vi "Read from Hardware.vi"(8 "error in":errorcluster, 10 "Values in":dbl[](array[numeric]), 11 "AIM ARINC-429 Rx Execution Unit in":refnum<class "Rx Execution Unit.lvclass">) -> (0 "error out":errorcluster, 2 "Values out":dbl[](array[numeric]), 3 "AIM ARINC-429 Rx Execution Unit out":refnum<class "Rx Execution Unit.lvclass">)   [LabVIEW 2020, in "AIM ARINC 429 Engine.lvlib" / "Implementation.lvlib" / "Rx Execution Unit.lvclass"]
uses:
  Rx Execution Unit.lvclass
  Execution Unit/Execution Unit.lvclass
  Hardware API/AIM ARINC 429 Hardware API.lvlib
  Custom Device/Custom Device.lvlib
  <instrlib>/AIM GmbH/ARINC-429/AIM429LV.lvlib
  C:/Git/niveristand-aim-arinc429-custom-device/Source/Custom Device Support/Engine/Implementation/Execution Unit/Execution Unit.lvclass
  C:/Git/niveristand-aim-arinc429-custom-device/Source/Custom Device Support/Engine/Interfaces/Execution Unit/Execution Unit.lvclass
  C:/Git/niveristand-aim-arinc429-custom-device/Source/Custom Device Support/Engine/Implementation/Rx Execution Unit/Rx Execution Unit.lvclass
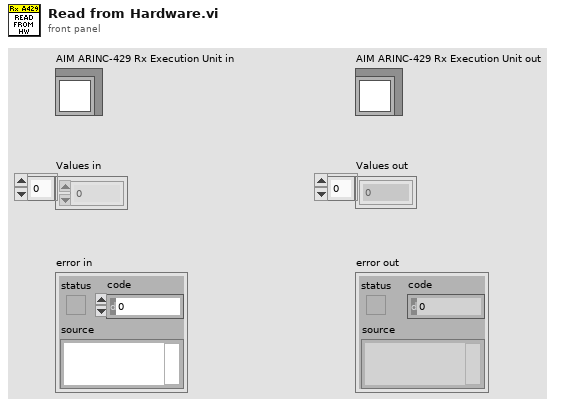
[diagram p1: front panel]
types:
  T1 = cluster{"hardware channel":u8, "label":u8, "SDI":u8}
  T2 = cluster{"gap":i16, "parity":i16, "long word":i16, "bit timing":i16, "timeout":i16}
  T3 = map{cluster{"hardware channel":u8, "label":u8, "SDI":u8}, cluster{"data word":u32, "time stamp":dbl}}
  T4 = typedef "AIM ARINC 429 Engine.lvlib/Custom Device.lvlib/Hardware Handles.ctl" = cluster{"module":u8}
  T5 = typedef "RT Hardware Channel Settings.ctl" = cluster{"channel #":u16, "channel handle":u64, "labels settings for RT":T6[]}
  T6 = typedef "RT Label Settings.ctl" = cluster{"Name":string, "xmlName":string, "label":T7, "transfer period":u32, "SDI_Enabled":bool, "SDI":u8, "parameter driver data":T8, "transfer type":T12, "has timestamp?":bool, "Label Disable/Trigger Channel Reference":T11, "Message Handle":u64, "Initialized?":bool, "Word Initial Raw Value":u32, "Label Timestamp Channel Data Reference":T13, "disabled":bool}
  T7 = typedef "Label.ctl" = u8
  T8 = typedef "RT Parameters.ctl" = cluster{"parameter definitions":T9[], "Tx parameter refs":T11[]}
  T9 = typedef "Parameter Definition.ctl" = cluster{"start index":i32, "size":i32, "encoding":T10, "signed":bool, "scale multiplier":dbl, "scale offset":dbl}
  T10 = typedef "Encoding and Decoding.lvlib/Encoding.ctl" = enum16{"BNR", "BCD", "Discrete"}
  T11 = typedef "Custom Device API.lvlib/Custom Device Item Ref.ctl" = u64
  T12 = typedef "Transfer Type.ctl" = enum16{"Scheduled", "Acyclic", "Block", "Strobe"}
  T13 = typedef "Custom Device API.lvlib/Data Reference.ctl" = i32
  T14 = cluster{"gap":bool, "parity":bool, "long word":bool, "bit timing":bool, "timeout":bool}
  T15 = typedef "Map of Identifiers to Indexes.ctl" = map{cluster{"Port":u8, "Label":u8, "SDI":u8}, cluster{"channel index":i32, "label index":i32, "start index":i32, "parameters":i32, "timestamp index":i32}}
  T16 = cluster{"receiving":T13, "specific errors":cluster{"gap":T13, "parity":T13, "long word ":T13, "bit timing":T13, "timeout":T13}}
  T17 = cluster{"receiving":dbl, "specific errors":cluster{"gap":dbl, "parity":dbl, "long word ":dbl, "bit timing":dbl, "timeout":dbl}}
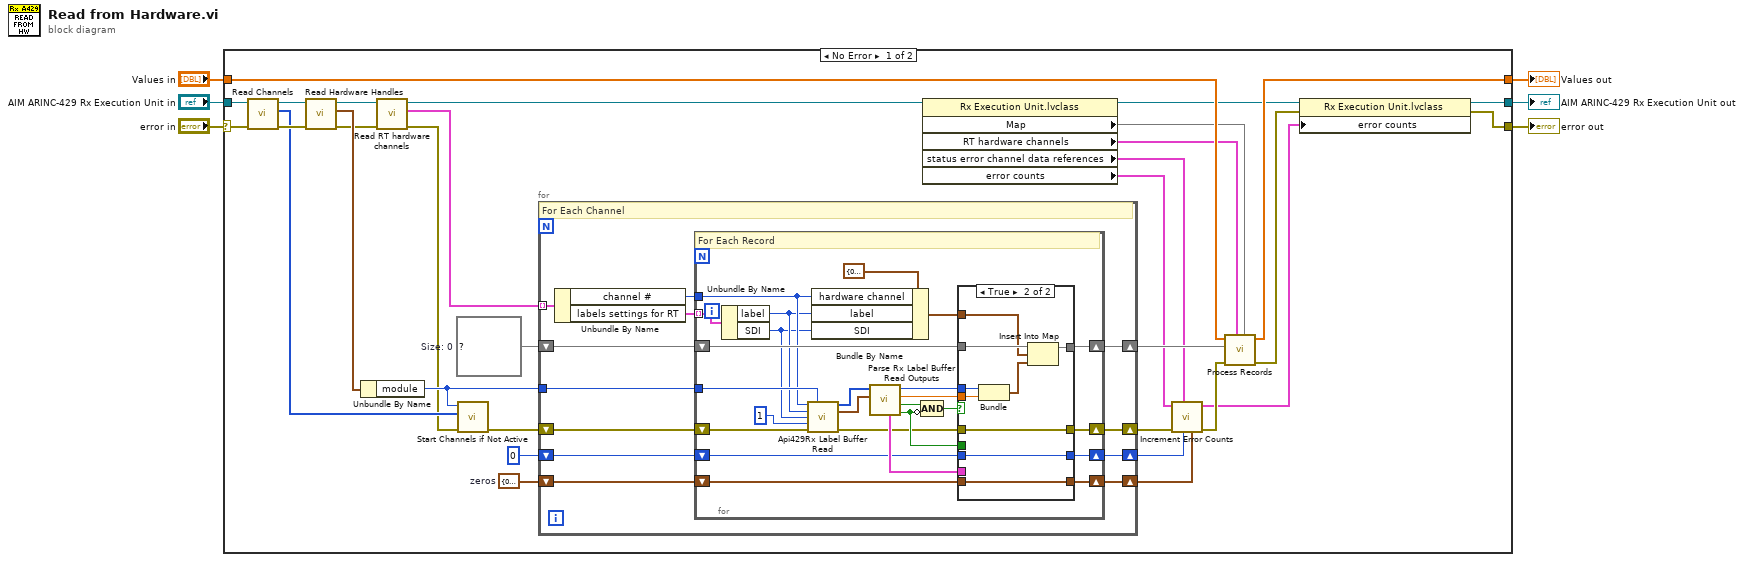
[diagram p0: block diagram]
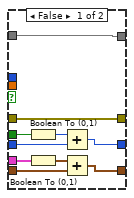
[diagram p2: hidden frame]
diagram:
  n1 = case shown="No Error" "error in" {
    selector: "error in" -> [w31 w96]
    tunnel: [w36 w97] -> w5
    tunnel: "AIM ARINC-429 Rx Execution Unit in" -> [w32 w97]
    tunnel: [w7 w96] -> w3
    tunnel: [w35 w95] -> w2
    tunnel: "Values in" -> [w34 w95]
    frame No Error {
      w16 = T2 {"gap"=0, "parity"=0, "long word"=0, "bit timing"=0, "timeout"=0}  # zeros
      w17 = T3 {}  # Size: 0
      n2 = call "Read Channels.vi"("error in"=w31, "execution unit in"=w32) -> ("error out"=w30:errorcluster, "channels"=w29:u8[], "execution unit out"=w33:refnum<class "Rx Execution Unit.lvclass">)  [unwired: 7 in]
      n3 = call "Read Hardware Handles.vi"("error in"=w30, "AIM ARINC-429 execution unit in"=w33) -> ("error out"=w11:errorcluster, "hardware handles"=w38:T4, "AIM ARINC-429 execution unit out"=w13:refnum<class "Rx Execution Unit.lvclass">)  [unwired: 7 in]
      n4 = Unbundle By Name(w38) -> ("module"=w14:u8)
      n5 = call "Read RT hardware channels.vi"("error in"=w11, "Rx execution unit in"=w13) -> ("error out"=w10:errorcluster, "RT hardware channels"=w9:T5[], "Rx execution unit out"=w12:refnum<class "Rx Execution Unit.lvclass">)  [unwired: 7 in]
      n6 = call "Start Channels if Not Active.vi"("error in"=w10, "channels"=w29, "module handle in"=w14) -> ("error out"=w37:errorcluster)  [unwired: 7 in, 1 out]
      n7 = for {
        tunnel: w14 -> [w42]
        shift-right: [w48] -> w25
        shift-left: w37 -> [w50]
        shift-right: [w46] -> w22
        shift-left: w16 -> [w44]
        shift-right: [w47] -> w23
        shift-left: i16 0 -> [w43]
        shift-right: [w49] -> w26
        shift-left: w17 -> [w45]
        tunnel: w9 -> [w41] mode=indexing
        # "For Each Channel"
        n8 = Unbundle By Name(w41) -> ("channel #"=w40:u16, "labels settings for RT"=w39:T6[])
        n9 = for {
          shift-right: [w68] -> w48
          shift-left: w50 -> [w62]
          shift-right: [w75] -> w49
          shift-left: w45 -> [w74]
          shift-right: [w73] -> w46
          shift-left: w44 -> [w72]
          shift-right: [w66] -> w47
          shift-left: w43 -> [w65]
          tunnel: w42 -> [w60]
          tunnel: w40 -> [w54]
          tunnel: w39 -> [w59] mode=indexing
          # "For Each Record"
          n10 = Unbundle By Name(w59) -> ("label"=w53:T7, "SDI"=w52:u8)
          n11 = call <instrlib>:"Api429Rx Label Buffer Read.vi"("b_Chn"=w54, "board_handle"=w60, "b_Label"=w53, "b_Sdi"=w52, "w_BufSize"=u16 1, "error in (no error)"=w62) -> ("px_LData out"=w57:u32[], "px_Info out"=w56:cluster{"ixw":u16, "inr":u16, "ci":u16}, "error out"=w61:errorcluster)  [unwired: 7 in]
          n12 = Bundle By Name(cluster=T1 {"hardware channel"=0, "label"=0, "SDI"=0} ("message info"), "hardware channel"=w54, "label"=w53, "SDI"=w52) -> (w51:T1)
          n13 = call "Parse Rx Label Buffer Read Outputs.vi"("px_Info out"=w56, "px_LData"=w57) -> ("receiving error"=w67:bool, "hit"=w70:bool, "time stamp"=w63:dbl, "data word"=w64:u32, "specific errors"=w71:T14)  [unwired: 5 in]
          n14 = Compound Arithmetic op=AND(w70, invert w67) -> (w69:bool)
          n15 = case shown="True" w69 {
            tunnel: w64 -> [_ w91]
            tunnel: w51 -> [_ w92]
            tunnel: [w85 w94] -> w75
            tunnel: w74 -> [w85 w93]
            tunnel: w72 -> [w83 w89]
            tunnel: [w79 w89] -> w73
            tunnel: w63 -> [_ w88]
            tunnel: w71 -> [w82 _]
            tunnel: w61 -> [w81 w87]
            tunnel: [w81 w87] -> w68
            tunnel: w67 -> [w80 _]
            tunnel: [w78 w86] -> w66
            tunnel: w65 -> [w76 w86]
            frame False {
              n16 = Boolean To (0,1)(Boolean=w80) -> (0, 1=w77:i16)
              n17 = Boolean To (0,1)(Boolean=w82) -> (0, 1=w84:T2)
              n18 = Add(x=w77, y=w76) -> (x+y=w78:i16)
              n19 = Add(x=w84, y=w83) -> (x+y=w79:T2)
            }
            frame True {
              n20 = Bundle("data word"=w91, "time stamp"=w88) -> (w90:cluster{"data word":u32, "time stamp":dbl})  [unwired: 1 in]
              n21 = Insert Into Map(map in=w93, key=w92, value=w90) -> (map out=w94:T3)  [unwired: 2 out]
            }
          }
        }
      }
      n22 = property class="Rx Execution Unit.lvclass"(reference=w12) -> (reference out=w18:refnum<class "Rx Execution Unit.lvclass">, "Map"=w28:T15, "RT hardware channels"=w27:T5[], "status error channel data references"=w21:T16, "error counts"=w20:T17)  [unwired: 1 in, 1 out]
      n23 = call "Increment Error Counts.vi"("specific errors"=w22, "receiving errors"=w23, "status error channel data references"=w21, "error in"=w25, "error counts"=w20) -> ("error out"=w24:errorcluster, "error counts"=w19:T17)  [unwired: 5 in]
      n24 = call "Process Records.vi"("map from message info to indexes"=w28, "RT hardware channel data"=w27, "error in"=w24, "map from message info to data word"=w26, "parameter values in"=w34) -> ("error out"=w8:errorcluster, "parameter values out"=w35:dbl[])  [unwired: 3 in]
      n25 = property class="Rx Execution Unit.lvclass"(reference=w18, error in=w8, "error counts"=w19) -> (reference out=w36:refnum<class "Rx Execution Unit.lvclass">, error out=w7:errorcluster)
    }
    frame Error {
    }
  }
  "error out" <- w3
  "AIM ARINC-429 Rx Execution Unit out" <- w5
  "Values out" <- w2
